vi "S7 TCP Test.vi"() -> ()   [LabVIEW 2011]
uses:
  S7 TCP API Library/S7 TCP.lvlib
panel:
  out "Comm Error":u16=33028
  in  "milliseconds to wait":u32=100
  in  "IP Address":string="192.168.1.2"
  in  "Data Block #":u16
  out "Loop Itteration":i32=16
  in  "Stop":bool
  out "Data Element 0 as Boolean array":bool[](array[boolean])
  in  "Read / Write":u8(ring)=5 items=["Read"=4, "Write"=5]
  in  "Address Areas":u8(ring)=131 items=["I/O (P)"=128, "Input (I)"=129, "Output (Q)"=130, "Bit Memory (M)"=131, "Data (DB)"=132, "Instance Data (DI)"=133, "Local Data (L)"=134, "Predecessor Local Data (VL)"=135]
  in  "Start Address (bytes)":u32=104
  out "Read Data":u8[](array[numeric])
  in  "Read Length (bytes)":u16=2
  in  "Write Data":u16=10000
  out "Data Valid":bool
  out "error out":errorcluster
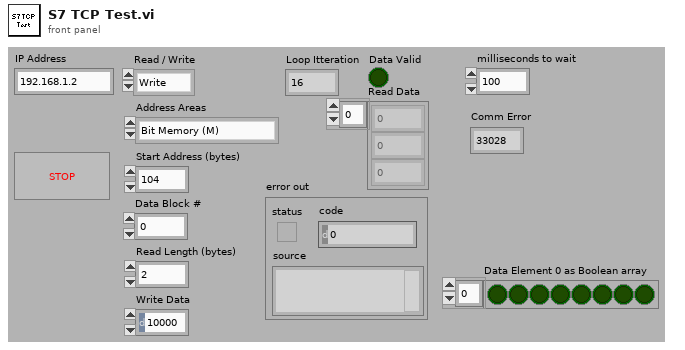
[diagram p1: front panel]
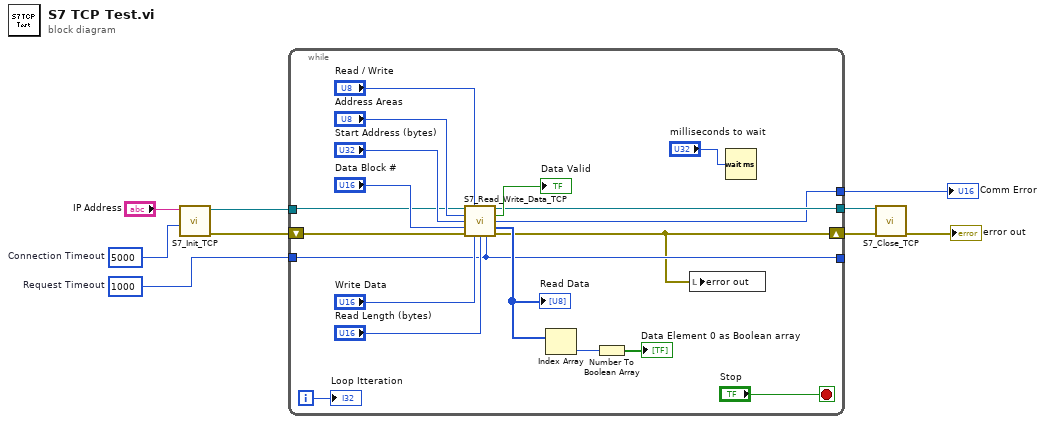
[diagram p0: block diagram]
diagram:
  w7 = u32 1000  # Request Timeout
  w8 = u32 5000  # Connection Timeout
  n1 = call "S7_Init_TCP.vi"("Connection Timeout"=w8, "IP Address"="IP Address") -> ("error out"=w4:errorcluster, "TCP Connection Ref"=w5:refnum<k5>)  [unwired: 3 in, 5 out]
  n2 = while {
    tunnel: w5 -> [w12]
    tunnel: w7 -> [w16]
    tunnel: [w16] -> _
    shift-right: [w13] -> w6
    shift-left: w4 -> [w23]
    tunnel: [w11] -> w2
    tunnel: [w10] -> w1
    i -> [w17]
    stop <- "Stop" stop-if-true
    n3 = call "S7_Read_Write_Data_TCP.vi"("TCP Connection Ref"=w12, "Read / Write"="Read / Write", "Address Areas"="Address Areas", "Start Address (bytes)"="Start Address (bytes)", "Data Block #"="Data Block #", "error in"=w23, "Write Data"="Write Data", "Length (bytes)"="Read Length (bytes)", "Timeout"=w16) -> ("TCP Connection Ref Out"=w11:refnum<k5>, "Data Valid"=→"Data Valid":bool, "Comm Error"=w10:u16, "Data Read"=w22:u8[], "error out"=w13:errorcluster)  [unwired: 1 in, 1 out]
    "Read Data" <- w22
    n4 = Index Array(array=w22) -> (element=w21:u8)  [unwired: 1 in]
    n5 = Number To Boolean Array(number=w21) -> (Boolean array=→"Data Element 0 as Boolean array":bool[])
    n6 = local write "error out"(w13) -> ()
    n7 = Wait (ms)(milliseconds to wait="milliseconds to wait") -> ()  [unwired: 1 out]
    "Loop Itteration" <- w17
  }
  "Comm Error" <- w1
  n8 = call "S7_Close_TCP.vi"("error in"=w6, "TCP Connection Ref"=w2) -> ("error out"=→"error out":errorcluster)  [unwired: 1 in, 8 out]
